vi "GetRunStatus.vi"(2 "error in (no error)":errorcluster, 3 "Timeout after N try (default = 100 (10 seconds))":i32=100) -> (0 "error out":errorcluster, 1 "Run Status":string)   [LabVIEW 2018, in "feGEM DataPacker.lvlib"]
uses:
  feGEM DataPacker.lvlib
  DataPacker/Utilities/PeriodicEnumTypeDef.ctl
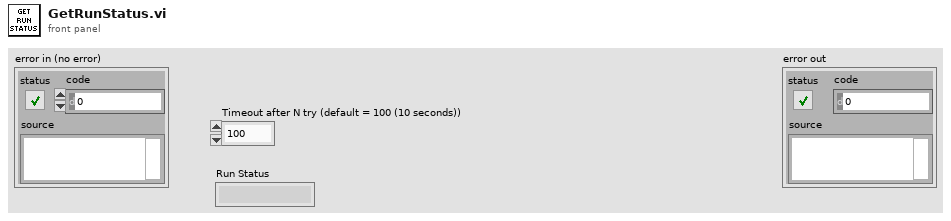
[diagram p1: front panel]
types:
  T1 = typedef "feGEM DataPacker.lvlib/PeriodicEnumTypeDef.ctl" = enum16{"GET_STATUS", "GET_HIST_RATE", "GET_RUNNO", "GET_RUN_START_T", "GET_RUN_STOP_T", "GET_TIME"}
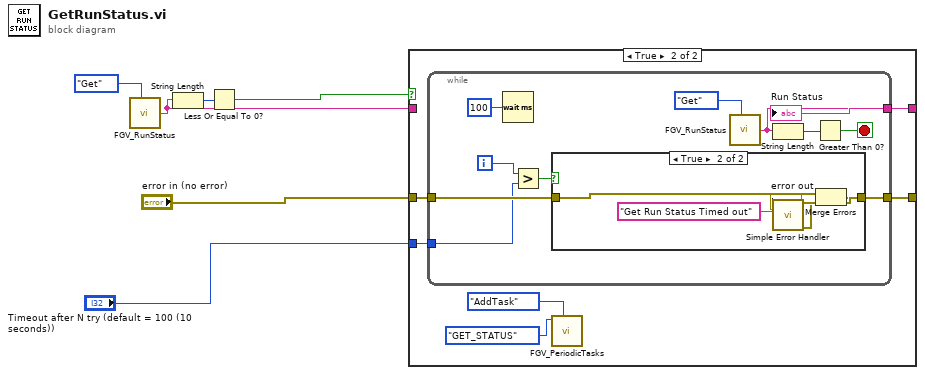
[diagram p0: block diagram]
diagram:
  n1 = call "FGV_RunStatus.vi"("Enum"=enum16{"Set", "Get"}."Get") -> ("Run Status"=w7:string)  [unwired: 4 in]
  n2 = String Length(string=w7) -> (length=w8:i32)
  n3 = Less Or Equal To 0?(x=w8) -> (x <= 0?=w5:bool)
  n4 = case shown="True" w5 {
    tunnel: [w10 w14] -> w6
    tunnel: w7 -> [w10 _]
    tunnel: "error in (no error)" -> [w9 w16]
    tunnel: [w9 w15] -> w3
    tunnel: "Timeout after N try (default = 100 (10 seconds))" -> [_ w11]
    frame False {
    }
    frame True {
      n5 = while {
        tunnel: w16 -> [w22]
        tunnel: [w21] -> w15
        tunnel: [w18] -> w14
        tunnel: w11 -> [w17]
        i -> [w24]
        stop <- w26 stop-if-true
        n6 = Wait (ms)(milliseconds to wait=u32 100) -> ()  [unwired: 1 out]
        n7 = Greater?(x=w24, y=w17) -> (0:w23:bool)
        n8 = case shown="True" w23 {
          tunnel: w22 -> [w27 w30]
          tunnel: [w27 w28] -> w21
          frame False {
          }
          frame True {
            n9 = call <vilib>:"Simple Error Handler.vi"("error source (\" \")"="Get Run Status Timed out" ("error source (\" \")")) -> ("error out"=w29:errorcluster)  [unwired: 4 in, 4 out]
            n10 = Merge Errors(w30, w29) -> (w28:errorcluster)
          }
        }
        n11 = call "FGV_RunStatus.vi"("Enum"=enum16{"Set", "Get"}."Get") -> ("Run Status"=w18:string)  [unwired: 4 in]
        n12 = String Length(string=w18) -> (length=w19:i32)
        n13 = Greater Than 0?(x=w19) -> (x > 0?=w26:bool)
      }
      n14 = call "FGV_PeriodicTasks.vi"("MIDAS Commands"=PeriodicEnumTypeDef."GET_STATUS" ("Enum"), "Task"=enum16{"AddTask", "GetTasks", "ClearTasks"}."AddTask" ("Enum 2")) -> ()  [unwired: 3 in, 1 out]
    }
  }
  "error out" <- w3
  "Run Status" <- w6
